vi "dvp Vi Get Noise Reduct3d.vi"(10 "pNoiseReduct3d":i32, 11 "handle":u32) -> (2 "pNoiseReduct3d out":i32, 3 "function return":u32(ring))   [LabVIEW 2018, in "LabViewDVPCamera.lvlib"]
doc: "LabviewDvp2Api dvpStatus dvpViGetNoiseReduct3d(dvpHandle handle, dvpInt32 *pNoiseReduct3d);"
uses:
  LabViewDVPCamera.lvlib
  LabViewDVPCamera/LabViewDVPCamera.dll
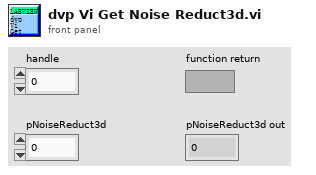
[diagram p1: front panel]
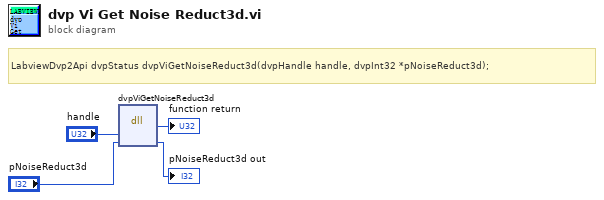
[diagram p0: block diagram]
diagram:
  # "LabviewDvp2Api dvpStatus dvpViGetNoiseReduct3d(dvpHandle handle, dvpInt32 *pNoiseReduct3d);"
  n1 = dll-call lib="C:/Program Files (x86)/DVP2 Labview cn 64/Sample/LabViewDVPCamera/LabViewDVPCamera.*" fn="dvpViGetNoiseReduct3d"("handle"="handle", "pNoiseReduct3d"="pNoiseReduct3d") -> (→"function return":u32, "pNoiseReduct3d"=→"pNoiseReduct3d out":i32)  [unwired: 4 in, 2 out]
